vi "Calculate Relative Path from Directory.vi"(8 "error in (no error)":errorcluster, 10 "path":path, 11 "directory":path) -> (0 "error out":errorcluster, 2 "relative path":path)   [LabVIEW 2021, in "MeasurementService Editor.lvlib"]
uses:
  MeasurementService Editor.lvlib
  <vilib>/Utility/error.llb/Error Cluster From Error Code.vi
  <vilib>/ErrorRing/Error Ring.xnode
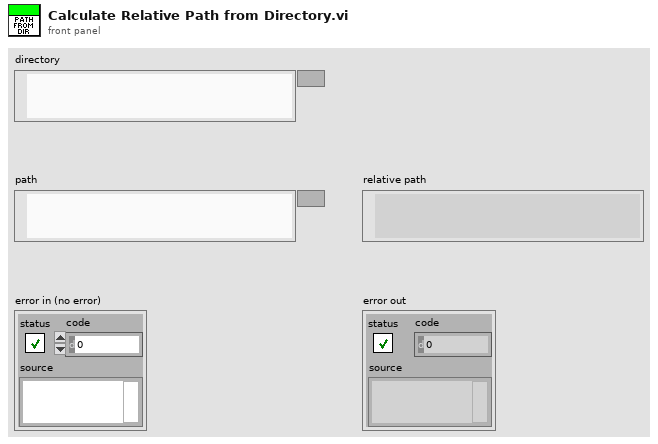
[diagram p1: front panel]
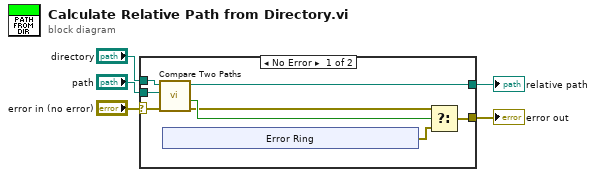
[diagram p0: block diagram]
diagram:
  n1 = case shown="No Error" "error in (no error)" {
    selector: "error in (no error)" -> [w6 w19]
    tunnel: "directory" -> [w13 _]
    tunnel: "path" -> [w12 _]
    tunnel: [w9 _] -> w3
    tunnel: [w8 w19] -> w2
    frame No Error {
      n2 = call <vilib>:"Compare Two Paths.vi"("error in (no error)"=w6, "Path 2"=w12, "Path 1"=w13) -> ("error out"=w10:errorcluster, "Path 2 Relative to Path 1?"=w11:bool, "Relative Path from 1 to 2"=w9:path)  [unwired: 5 in, 1 out]
      n3 = xnode "Error Ring"() -> ("error out"=w7:errorcluster)
      n4 = Select(t=w10, s=w11, f=w7) -> (s? t:f=w8:errorcluster)
    }
    frame Error {
    }
  }
  "error out" <- w2
  "relative path" <- w3
